vi "Script Msg Private Data.vi"(6 "PD Cluster":refnum<vi>, 8 "error in":errorcluster, 9 "PD Control":refnum<vi>, 10 "Terminal Attributes (Init Msg Input)":T1) -> (0 "error out":errorcluster)   [LabVIEW 2025, in "_Rescript.lvlib" / "Msg.lvlib" / "Msg.lvclass"]
uses:
  Msg.lvclass
  Terminal Attributes.ctl
  Attributes.ctl
  _Rescript.lvlib
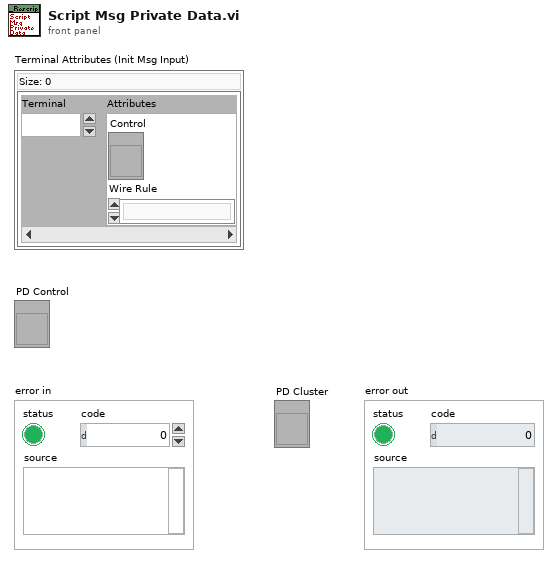
[diagram p1: front panel]
types:
  T1 = typedef "_Rescript.lvlib/Terminal Attributes.ctl" = map{i32, T2}
  T2 = typedef "_Rescript.lvlib/Attributes.ctl" = cluster{"Control":refnum<vi>, "Wire Rule":enum16{"Invalid Wire Rule", "Required", "Recommended", "Optional", "Dynamic Dispatch"}}
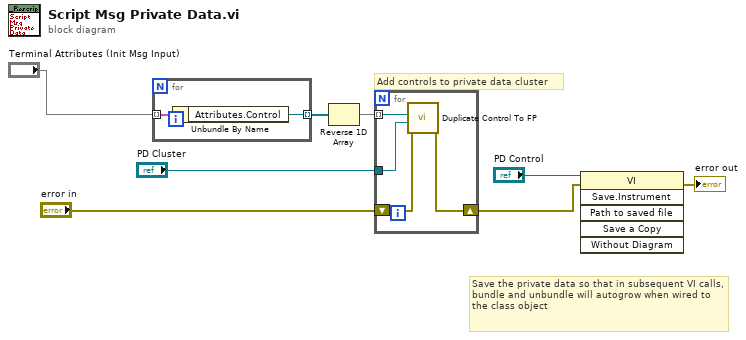
[diagram p0: block diagram]
diagram:
  # "Add controls to private data cluster"
  # "Save the private data so that in subsequent VI calls, bundle and unbundle will autogrow when wired to the class object"
  n1 = for {
    tunnel: "Terminal Attributes (Init Msg Input)" -> [w10] mode=indexing
    tunnel: [w9] -> w8 mode=indexing
    n2 = Unbundle By Name(w10) -> ("Attributes.Control"=w9:refnum<vi>)
  }
  n3 = Reverse 1D Array(array=w8) -> (reversed array=w7:refnum<vi>[])
  n4 = for {
    tunnel: "PD Cluster" -> [w12]
    shift-right: [w13] -> w6
    shift-left: "error in" -> [w14]
    tunnel: w7 -> [w11] mode=indexing
    n5 = call "Duplicate Control To FP.vi"("error in"=w14, "Owner"=w12, "Control"=w11) -> ("error out"=w13:errorcluster)  [unwired: 8 in]
  }
  n6 = invoke class="VI" method="Save.Instrument"(reference="PD Control", error in=w6) -> (error out=→"error out":errorcluster)  [unwired: 4 in, 5 out]
